vi "Close.vi"(8 "Error in":errorcluster caption="Error in (no error)", 11 "DVR":T1) -> (0 "Error out":errorcluster, 3 "DVR(dup)":T1)   [LabVIEW 2020, in "DVR-Module.lvlib"]
uses:
  DVR-Module.lvlib
  DVR.ctl
  DataDef.ctl
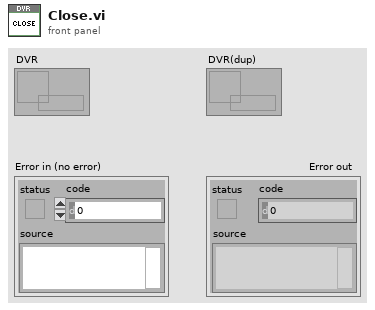
[diagram p1: front panel]
types:
  T1 = typedef "DVR-Module.lvlib/DVR.ctl" = refnum<data-value>
  T2 = typedef "DataDef.ctl" = cluster{"dbl":dbl}
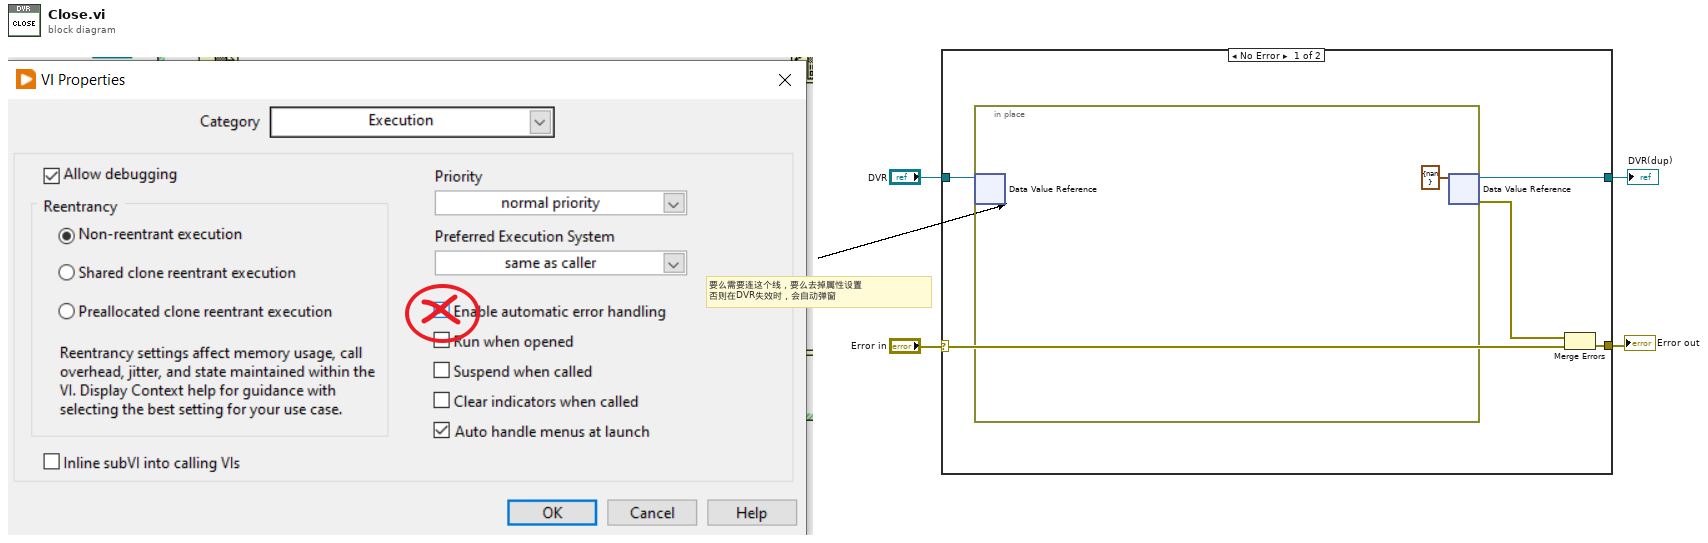
[diagram p0: block diagram]
diagram:
  # "要么需要连这个线，要么去掉属性设置\n否则在DVR失效时，会自动弹窗"
  n1 = case shown="No Error" "Error in" {
    selector: "Error in" -> [w5 w12]
    tunnel: "DVR" -> [w9 w11]
    tunnel: [w8 w11] -> w3
    tunnel: [w7 w12] -> w2
    frame No Error {
      n2 = in-place {
        n3 = in-place-dvr #1(w9) -> ()  [unwired: 2 out]
        n4 = in-place-dvr #1(T2 {"dbl"=nan} ("data value")) -> (w8:T1, w6:errorcluster)
      }
      n5 = Merge Errors(w6, w5) -> (w7:errorcluster)
    }
    frame Error {
    }
  }
  "Error out" <- w2
  "DVR(dup)" <- w3
